vi "Destroy.vi"(8 "Error In":errorcluster, 11 "reference in":refnum<class "TextDecorator.lvclass">) -> (0 "Error Out":errorcluster, 3 "reference out":refnum<class "TextDecorator.lvclass">)   [LabVIEW 2024, in "TextDecorator.lvclass"]
uses:
  TextDecorator.lvclass
  TextDecorator.lvclass/TextDecorator.ctl
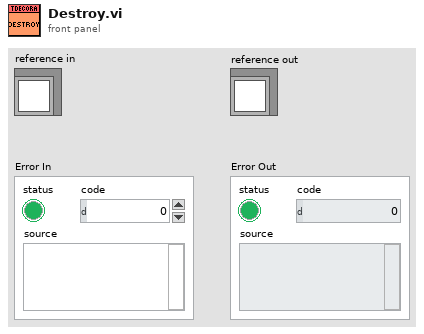
[diagram p1: front panel]
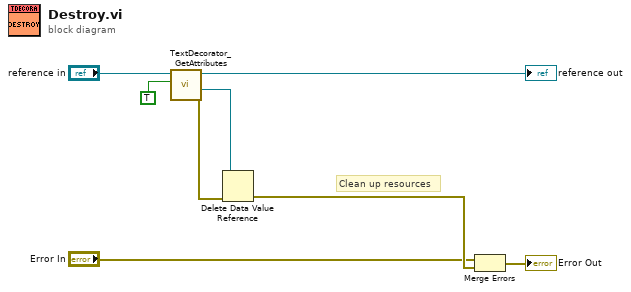
[diagram p0: block diagram]
diagram:
  # "Clean up resources"
  n1 = call "TextDecorator_GetAttributes.vi"("OnlyGetDvrReference(False)"=TRUE, "reference in"="reference in") -> ("Error Out"=w5:errorcluster, "DataRef"=w4:refnum<data-value>, "reference out"=→"reference out":refnum<class "TextDecorator.lvclass">)  [unwired: 6 in, 1 out]
  n2 = Delete Data Value Reference(data value reference=w4, error in=w5) -> (error out=w3:errorcluster)  [unwired: 1 out]
  n3 = Merge Errors("Error In", w3) -> (→"Error Out":errorcluster)
